vi "TCP AK-LNI Warnung filtern.vi"(11 "error in (no error)":errorcluster caption="Fehler (Eingang, kein Fehler)") -> (3 "error out":errorcluster caption="Fehler (Ausgang)")   [LabVIEW 2020, in "Linearisierung v2.lvlib" / "Gasteiler.lvlib" / "AK Komm Gasteiler.lvlib"]
doc: "Entfernt die Warnung, die dadurch entsteht, dass in VISA-Lesen mehr Bytes angefordert werden, als dann empfangen werden.\n( Der Lesevorgang wird durch den \"Termination Character\" KORREKT abgebrochen. )\n\nDie Warnung:\nVISA: (Hex 0x3FFF0006) Es wurden weniger Bytes übertragen als angefordert. Möglicherweise sind noch weitere Daten verfügbar."
uses:
  AK Komm Gasteiler.lvlib
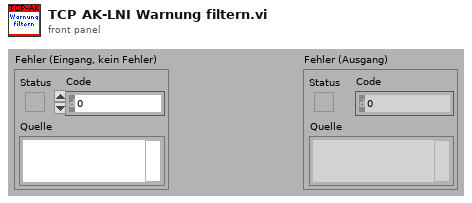
[diagram p1: front panel]
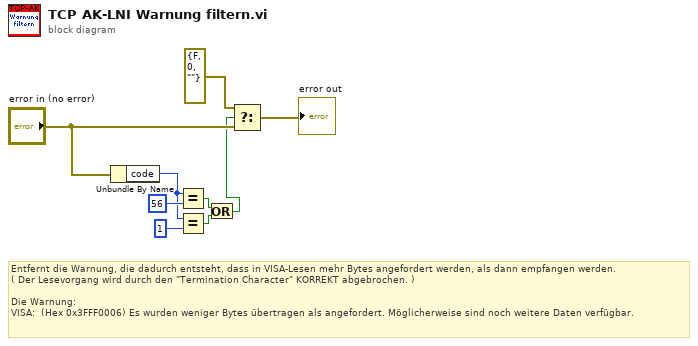
[diagram p0: block diagram]
diagram:
  # "Entfernt die Warnung, die dadurch entsteht, dass in VISA-Lesen mehr Bytes angefordert werden, als dann empfangen werden.\n( Der Lesevorgang wird durch den \"Termination Character\" KORREKT abgebrochen. )\n\nDie Warnung:\nVISA:  (Hex 0x3FFF0006) Es wurden weniger Bytes übertragen als angefordert. Möglicherweise sind noch weitere Daten verfügbar."
  n1 = Unbundle By Name("error in (no error)") -> ("code"=w4:i32)
  n2 = Equal?(x=w4, y=56) -> (x = y?=w2:bool)
  n3 = Equal?(x=w4, y=1) -> (x = y?=w3:bool)
  n4 = Or(x=w2, y=w3) -> (x .or. y?=w1:bool)
  n5 = Select(t=errorcluster {"status"=FALSE, "code"=0, "source"=""} ("error in (no error)"), s=w1, f="error in (no error)") -> (s? t:f=→"error out":errorcluster)
